vi "Kinect Controler.vi"() -> ()   [LabVIEW 2015]
uses:
  subVIs/Video Resolution Control.ctl
  subVIs/Video Format Control.ctl
  subVIs/Depth Format Control.ctl
  subVIs/Depth Resolution Control.ctl
  subVIs/Led Control.ctl
  subVIs/Log Level Control.ctl
  <vilib>/myRIO/Instrument Drivers/Onboard Devices/Accelerometer/typedefs/Accelerometer Reference.ctl
  <vilib>/myRIO/Common/Instrument Driver Framework/Utilities/typedefs/myRIO Generic Hardware Reference.ctl
  <vilib>/myRIO/Common/Instrument Driver Framework/Utilities/typedefs/Hardware Version Enum.ctl
  <vilib>/myRIO/Common/Instrument Driver Framework/Utilities/typedefs/myRIO v1.0 Reference.ctl
  <vilib>/myRIO/Common/Instrument Driver Framework/Utilities/typedefs/Generic FPGA Reference.ctl
  <vilib>/myRIO/Common/Instrument Driver Framework/myRIO v1.0/Accelerometer/typedefs/Accelerometer Channels List.ctl
  <vilib>/myRIO/Common/Instrument Driver Framework/myRIO v1.0/Accelerometer/typedefs/Accelerometer Channels Enum.ctl
  <vilib>/userdefined/High Color/nirio_resource_hc.ctl
  <vilib>/myRIO/Common/Instrument Driver Framework/Utilities/vis/Is FPGA Ref Available.vi
  <vilib>/myRIO/Common/Instrument Driver Framework/myRIO v1.0/Accelerometer/vis/myRIO v1.1 Open Accelerometer.vi
  <vilib>/myRIO/Instrument Drivers/Onboard Devices/Accelerometer/vis/Read.vi
  <vilib>/myRIO/Common/Instrument Driver Framework/Utilities/vis/Validate Channels.vi
  <vilib>/myRIO/Common/Instrument Driver Framework/myRIO v1.0/Accelerometer/vis/myRIO v1.0 Reserve Accelerometer.vi
  <vilib>/myRIO/Common/Instrument Driver Framework/myRIO v1.0/UART/vis/myRIO v1.0 Close UART.vi
  <vilib>/myRIO/Common/Instrument Driver Framework/myRIO v1.0/Resource Manager/vis/myRIO v1.0 Reserve Channel List.vi
  <vilib>/myRIO/Common/Instrument Driver Framework/myRIO v1.0/Accelerometer/vis/myRIO v1.0 Build MUX Configuration Accelerometer.vi
  <vilib>/myRIO/Common/Instrument Driver Framework/myRIO v1.0/Resource Manager/vis/myRIO v1.0 Reserve Channel.vi
  <vilib>/myRIO/Common/Instrument Driver Framework/myRIO v1.0/Resource Manager/vis/myRIO v1.0 Unreserve Channel.vi
  <vilib>/myRIO/Common/Instrument Driver Framework/myRIO v1.0/Resource Manager/vis/myRIO v1.0 Build Mutex Name.vi
  <vilib>/Utility/VariantDataType/GetNumericInfo.vi
  <vilib>/Utility/error.llb/Error Cluster From Error Code.vi
  <vilib>/myRIO/Common/Instrument Driver Framework/myRIO v1.0/myRIO v1.1 Open.vi
  <vilib>/myRIO/Common/Instrument Driver Framework/myRIO v1.0/Accelerometer/vis/myRIO v1.0 Get Scaling Constant Accelerometer.vi
  <vilib>/myRIO/Common/Instrument Driver Framework/Utilities/vis/IO Manager.vi
  <vilib>/myRIO/Common/Instrument Driver Framework/Utilities/vis/Configuration Manager.vi
  <vilib>/myRIO/Common/Instrument Driver Framework/myRIO v1.0/myRIO v1.0 Close.vi
  <vilib>/myRIO/Common/Instrument Driver Framework/myRIO v1.0/Accelerometer/vis/myRIO v1.0 Read Accelerometer.vi
  <vilib>/myRIO/Common/Instrument Driver Framework/Utilities/vis/FPGA Ref Manager.vi
  <vilib>/myRIO/Common/Instrument Driver Framework/myRIO v1.0/myRIO v1.0 Reset FPGA.vi
  <vilib>/myRIO/Common/Instrument Driver Framework/myRIO v1.0/IRQ/vis/myRIO v1.0 IRQ Info FGV.vi
  <vilib>/myRIO/Common/Instrument Driver Framework/myRIO v1.0/IRQ/vis/myRIO v1.0 Timer IRQ Info FGV.vi
  <vilib>/myRIO/Common/Instrument Driver Framework/myRIO v1.0/IRQ/vis/myRIO v1.0 ISR Agent.vi
  <vilib>/myRIO/Express VI/Onboard Devices/Accelerometer/Accelerometer Express VI.xnode
  <vilib>/myRIO/Instrument Drivers/Onboard Devices/Accelerometer/vis/myRIO Accelerometer Open.xnode
  <vilib>/myRIO/Instrument Drivers/Utilities/Utilities.lvlib
  <vilib>/myRIO/Instrument Drivers/Onboard Devices/Accelerometer/Accelerometer.lvlib
panel:
  out "error out 3":errorcluster
  out "Video":picture
  out "error out 2":errorcluster
  out "Acceleration":T1(graph)
  out "error out":errorcluster
  in  "Led Option":T2=enum."LED_RED"
  in  "Video & Depth Config":T7
  in  "Tilt degree":i32=5 min=-28 max=28
  in  "stop":bool
  out "Depth image":picture
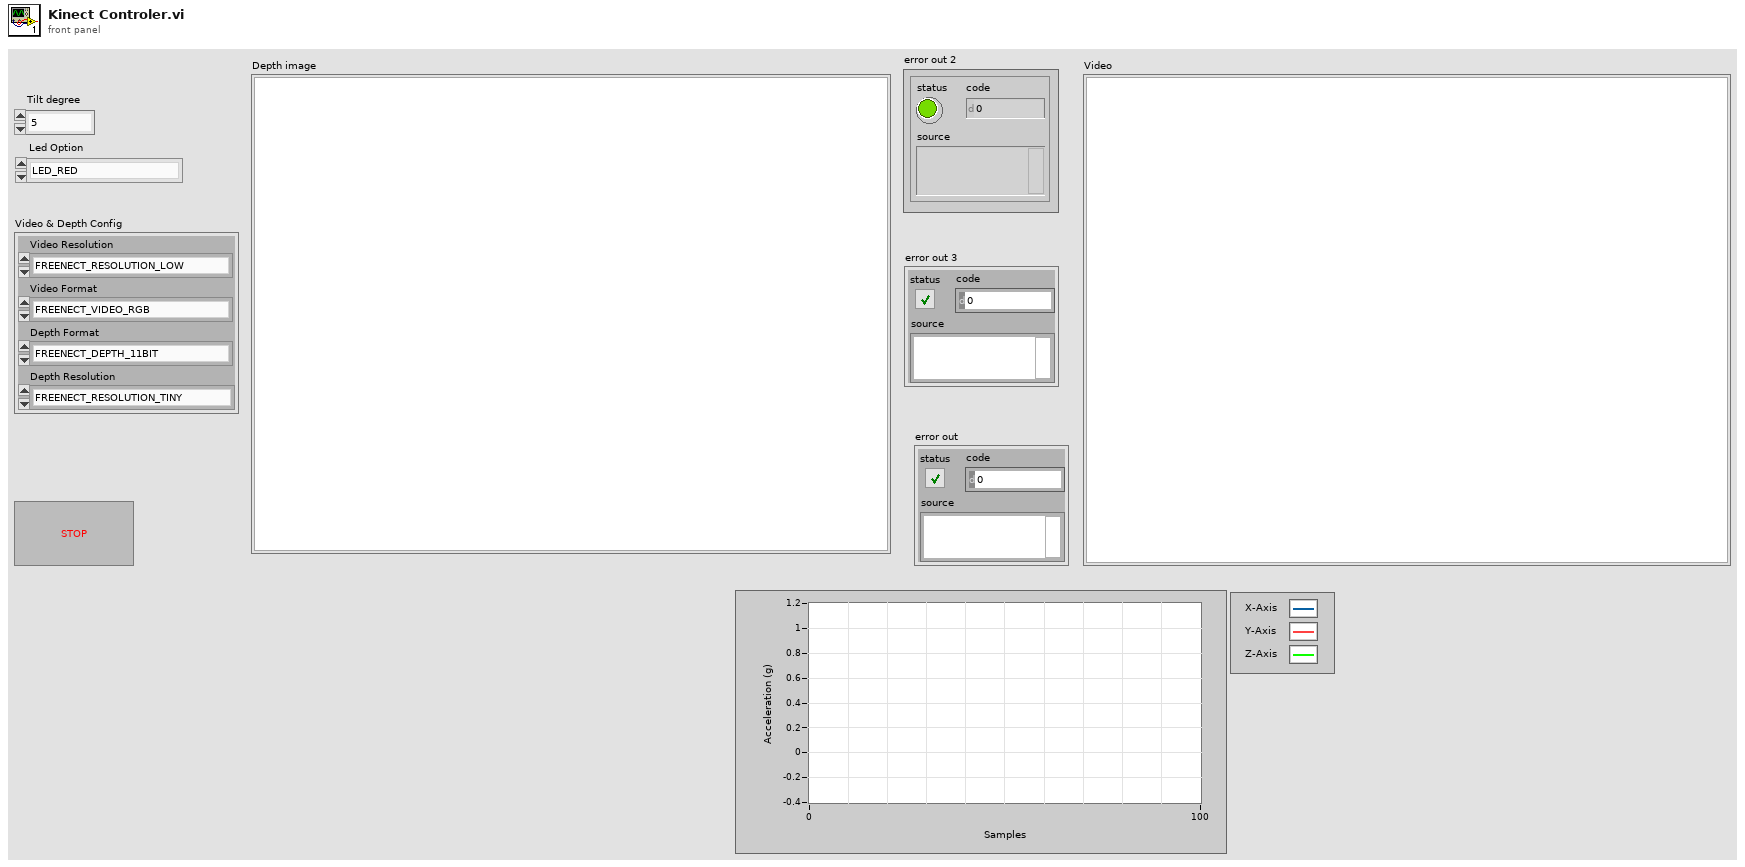
[diagram p1: front panel]
types:
  T1 = cluster{"X-Axis":dbl, "Y-Axis":dbl, "Z-Axis":dbl}
  T2 = typedef "Led Control.ctl" = enum32{"LED_OFF", "LED_GREEN", "LED_RED", "LED_YELLOW", "LED_BLINK_GREEN", "LED_BLINK_GREEN2", "LED_BLINK_RED_YELLOW"}
  T3 = typedef "Video Resolution Control.ctl" = enum32{"FREENECT_RESOLUTION_LOW", "FREENECT_RESOLUTION_MEDIUM", "FREENECT_RESOLUTION_HIGH"}
  T4 = typedef "Video Format Control.ctl" = enum32{"FREENECT_VIDEO_RGB", "FREENECT_VIDEO_BAYER", "FREENECT_VIDEO_IR_8BIT", "FREENECT_VIDEO_IR_10BIT", "FREENECT_VIDEO_IR_10BIT_PACKED", "FREENECT_VIDEO_YUV_RGB", "FREENECT_VIDEO_YUV_RAW"}
  T5 = typedef "Depth Format Control.ctl" = enum32{"FREENECT_DEPTH_11BIT", "FREENECT_DEPTH_10BIT", "FREENECT_DEPTH_11BIT_PACKED", "FREENECT_DEPTH_10BIT_PACKED", "FREENECT_DEPTH_REGISTERED", "FREENECT_DEPTH_MM"}
  T6 = typedef "Depth Resolution Control.ctl" = enum16{"FREENECT_RESOLUTION_TINY", "FREENECT_RESOLUTION_LOW", "FREENECT_RESOLUTION_MEDIUM"}
  T7 = cluster{"Video Resolution":T3, "Video Format":T4, "Depth Format":T5, "Depth Resolution":T6}
  T8 = typedef "Log Level Control.ctl" = enum32{"FREENECT_LOG_FATAL", "FREENECT_LOG_ERROR", "FREENECT_LOG_WARNING", "FREENECT_LOG_NOTICE", "FREENECT_LOG_INFO", "FREENECT_LOG_DEBUG", "FREENECT_LOG_SPEW", "FREENECT_LOG_FLOOD"}
  T9 = typedef "Accelerometer.lvlib/Accelerometer Reference.ctl" = cluster{"myRIO Reference":T10, "Accelerometer Channels List":T14, "LSB Weight":dbl}
  T10 = typedef "myRIO Generic Hardware Reference.ctl" = cluster{"myRIO Model":T11, "myRIO Hardware Reference":T12}
  T11 = typedef "Hardware Version Enum.ctl" = enum16{"Unknown", "myRIO-1900", "myRIO-1950", "roboRIO"}
  T12 = typedef "myRIO v1.0 Reference.ctl" = cluster{"Generic FPGA Reference":T13, "Allow multiple opens":bool}
  T13 = typedef "Generic FPGA Reference.ctl" = refnum<k20>
  T14 = typedef "Accelerometer Channels List.ctl" = T15[]
  T15 = typedef "Accelerometer Channels Enum.ctl" = enum16{"Not Connected", "X-Axis", "Y-Axis", "Z-Axis"}
  T16 = typedef "nirio_resource_hc.ctl" = tag
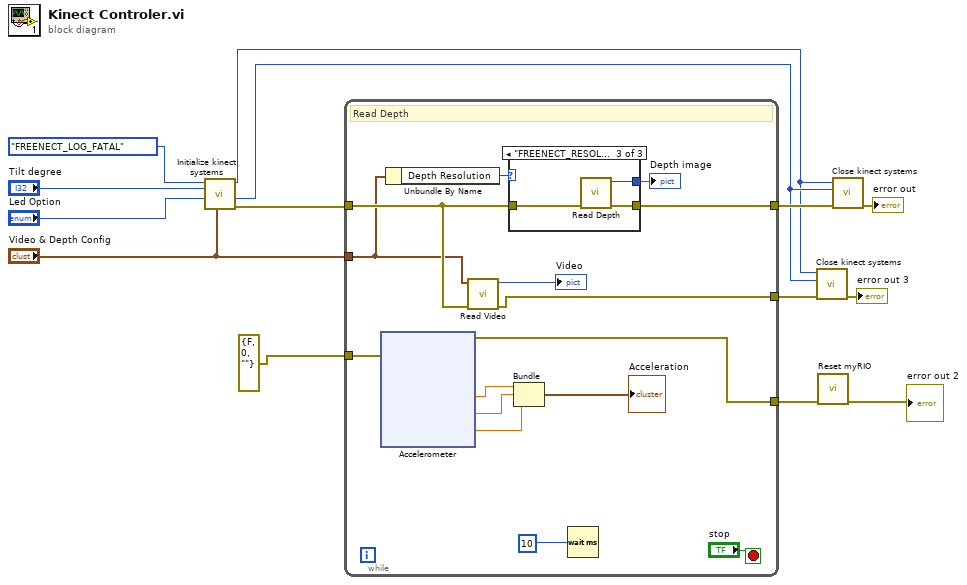
[diagram p0: block diagram]
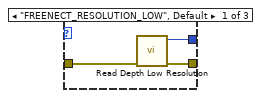
[diagram p2: hidden frame]
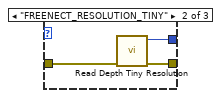
[diagram p3: hidden frame]
diagram:
  n1 = call "Initialize kinect systems.vi"("Video and Depth config"="Video & Depth Config", "Led Option"="Led Option", "tilt degree"="Tilt degree", "Log Level"=Log_Level_Control."FREENECT_LOG_FATAL") -> ("error out"=w13:errorcluster, "Kinect Handle"=w4:i64, "Video Handle out"=w3:i64)  [unwired: 4 in, 1 out]
  n2 = while {
    tunnel: w13 -> [w23]
    tunnel: [w27] -> w14
    tunnel: "Video & Depth Config" -> [w22]
    tunnel: [w21] -> w5
    tunnel: errorcluster {"status"=FALSE, "code"=0, "source"=""} ("error in (no error)") -> [w16]
    tunnel: [w15] -> w1
    stop <- "stop" stop-if-true
    # "Read Depth"
    n3 = xnode "Accelerometer"("error in (no error)"=w16) -> ("X-Axis"=w19:dbl, "Y-Axis"=w18:dbl, "Z-Axis"=w17:dbl, "error out"=w15:errorcluster)
    n4 = Unbundle By Name(w22) -> ("Depth Resolution"=w25:T6)
    n5 = call "Read Video.vi"("error in (no error)"=w23, "input cluster"=w22) -> ("error out"=w21:errorcluster, "RGB image"=→"Video":picture)  [unwired: 7 in, 1 out]
    n6 = case shown="\"FREENECT_RESOLUTION_MEDIUM\"" w25 {
      tunnel: w23 -> [w71 w72 w77]
      tunnel: [w70 w73 w76] -> w27
      tunnel: [w69 w74 w75] -> w26
      frame "FREENECT_RESOLUTION_LOW", Default {
        n7 = call "Read Depth Low Resolution.vi"("error in (no error)"=w71) -> ("error out"=w70:errorcluster, "Depth image"=w69:picture)  [unwired: 9 in]
      }
      frame "FREENECT_RESOLUTION_TINY" {
        n8 = call "Read Depth Tiny Resolution.vi"("error in (no error)"=w72) -> ("error out"=w73:errorcluster, "Depth image"=w74:picture)  [unwired: 9 in]
      }
      frame "FREENECT_RESOLUTION_MEDIUM" {
        n9 = call "Read Depth.vi"("error in (no error)"=w77) -> ("error out"=w76:errorcluster, "Depth image"=w75:picture)  [unwired: 9 in]
      }
    }
    "Depth image" <- w26
    n10 = Bundle("X-Axis"=w19, "Y-Axis"=w18, "Z-Axis"=w17) -> (→"Acceleration":T1)  [unwired: 1 in]
    n11 = Wait (ms)(milliseconds to wait=u32 10) -> ()  [unwired: 1 out]
  }
  n12 = call "Close kinect systems.vi"("error in (no error)"=w5, "Kinect Handle"=w4, "Video handle in"=w3) -> ("error out"=→"error out 3":errorcluster)  [unwired: 8 in]
  n13 = call <vilib>:"Reset myRIO.vi"("error in (no error)"=w1) -> ("error out"=→"error out 2":errorcluster)  [unwired: 10 in]
  n14 = call "Close kinect systems.vi"("error in (no error)"=w14, "Kinect Handle"=w4, "Video handle in"=w3) -> ("error out"=→"error out":errorcluster)  [unwired: 8 in]
